vi "Write Peaks.vi"(8 "error in (no error)":errorcluster, 10 "Peaks":T1={"Amplitude"=1000.0, "Center"=694.3, "Width"=0.4} {"Width" format="%#_gnm"; "Center" format="%#_gnm"}, 11 "Spectrometer Driver in":refnum<class "Spectrometer Driver.lvclass">) -> (0 "error out":errorcluster, 3 "Spectrometer Driver out":refnum<class "Spectrometer Driver.lvclass">)   [LabVIEW 2019, in "Spectrometer Driver.lvclass"]
uses:
  Spectrometer Driver.lvclass
  Utilities/Fit/Peak Parameters.ctl
  Spectrometer Driver.lvclass/Spectrometer Driver.ctl
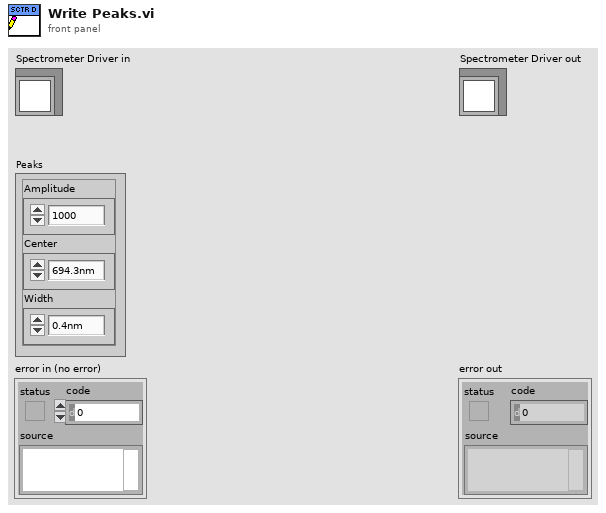
[diagram p1: front panel]
types:
  T1 = typedef "Peak Parameters.ctl" = cluster{"Amplitude":dbl, "Center":dbl, "Width":dbl}
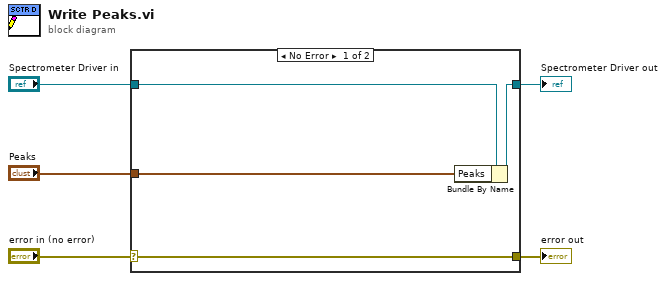
[diagram p0: block diagram]
diagram:
  n1 = case shown="No Error" "error in (no error)" {
    selector: "error in (no error)" -> [w9 w10]
    tunnel: [w9 w10] -> w4
    tunnel: [w7 w11] -> w2
    tunnel: "Spectrometer Driver in" -> [w8 w11]
    tunnel: "Peaks" -> [w6 _]
    frame No Error {
      n2 = Bundle By Name(cluster=w8, "Peaks"=w6) -> (w7:refnum<class "Spectrometer Driver.lvclass">)
    }
    frame Error {
    }
  }
  "error out" <- w4
  "Spectrometer Driver out" <- w2
